vi "WPI_ADI_IMU_Get Instant.vi"(8 "error in":errorcluster, 11 "ADI IMU Interrupt DevRef":T1={"SimpleGyroDevRef"={"DevStatus"={"status"=FALSE, "code"=0, "source"=""}, "Handle"=0, "SPI Bus"=enum."SPI On-Board, CS0", "Device Found"=FALSE, "Sample Rate"=0.0, "Device Ready"=FALSE, "Yaw Axis"=enum."Z", "AHRS Algorithm"=enum."Complementary"}, "InterruptRef"={"DevStatus"={"status"=FALSE, "code"=0, "source"=""}, "InterruptIndex"=enum."0"}} {"SimpleGyroDevRef"."Sample Rate" min=0.25 max=100.0 step=0.25}) -> (0 "error out":errorcluster, 1 "Sensor Ready Out":bool, 2 "IMU Data":T6, 3 "ADI IMU DevRef":T2={"DevStatus"={"status"=FALSE, "code"=0, "source"=""}, "Handle"=0, "SPI Bus"=enum."SPI On-Board, CS0", "Device Found"=FALSE, "Sample Rate"=0.0, "Device Ready"=FALSE, "Yaw Axis"=enum."Z", "AHRS Algorithm"=enum."Complementary"} {"Sample Rate" min=0.25 max=100.0 step=0.25})   [LabVIEW 2015, in "FRC ADI MXP IMU.lvlib"]
doc: "Get instantaneous readings from the Analog Devices MXP IMU board (Gyro Rate, Accel, Magnetometer, Barometer, Temp). This requires that the IMU_Loop VI be located in Periodic Tasks."
uses:
  FRC ADI MXP IMU.lvlib
  WPI_AnalogDevicesIMUDevRef.ctl
  <vilib>/Rock Robotics/SystemInterfaces/spilib/spi_bus.ctl
  WPI_AnalogDevicesIMUInterruptDevRef.ctl
  <vilib>/Rock Robotics/WPI/Interrupt/WPI_InterruptRef.ctl
  <vilib>/Rock Robotics/SystemInterfaces/Interrupt/FPGA_InterruptIndex.ctl
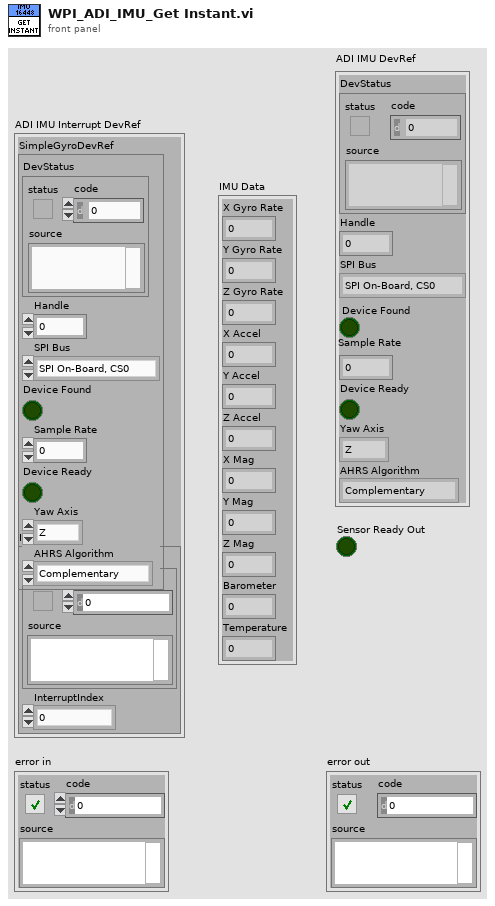
[diagram p1: front panel]
types:
  T1 = typedef "FRC ADI MXP IMU.lvlib/WPI_AnalogDevicesIMUInterruptDevRef.ctl" = cluster{"SimpleGyroDevRef":T2, "InterruptRef":T4}
  T2 = typedef "FRC ADI MXP IMU.lvlib/WPI_AnalogDevicesIMUDevRef.ctl" = cluster{"DevStatus":errorcluster, "Handle":i32, "SPI Bus":T3, "Device Found":bool, "Sample Rate":dbl, "Device Ready":bool, "Yaw Axis":enum16{"X", "Y", "Z"}, "AHRS Algorithm":enum16{"Complementary", "Madgwick"}}
  T3 = typedef "spi_bus.ctl" = enum16{"SPI On-Board, CS0", "SPI On-Board, CS1", "SPI On-Board, CS2", "SPI On-Board, CS3", "SPI MXP", "Invalid"}
  T4 = typedef "WPI_InterruptRef.ctl" = cluster{"DevStatus":errorcluster, "InterruptIndex":T5}
  T5 = typedef "FPGA_InterruptIndex.ctl" = enum8{"0", "1", "2", "3", "4", "5", "6", "7", "Invalid"}
  T6 = cluster{"X Gyro Rate":dbl, "Y Gyro Rate":dbl, "Z Gyro Rate":dbl, "X Accel":dbl, "Y Accel":dbl, "Z Accel":dbl, "X Mag":dbl, "Y Mag":dbl, "Z Mag":dbl, "Barometer":dbl, "Temperature":dbl}
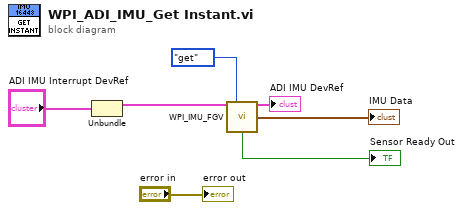
[diagram p0: block diagram]
diagram:
  n1 = Unbundle("ADI IMU Interrupt DevRef") -> ("SimpleGyroDevRef"=w3:T2)  [unwired: 1 out]
  n2 = call "WPI_IMU_FGV.vi"("SimpleGyroDevRef"=w3, "Operation"=enum16{"set", "get"}."get") -> ("SimpleGyroDevRef"=→"ADI IMU DevRef":T2, "IMU Data Out"=→"IMU Data":T6, "Sensor Ready Out"=→"Sensor Ready Out":bool)  [unwired: 7 in, 4 out]
  "error out" <- "error in"
